vi "SaveData.vi"(1 "output cluster":cluster{"Position":dbl, "data":dbl[][]}, 3 "File name":string="radial.txt", 4 "File path":path=path "C:/Documents and Settings/Administrator/Desktop/labview/M_Coupling/radial_coupling") -> ()   [LabVIEW 2013]
panel:
  out "appended path":path
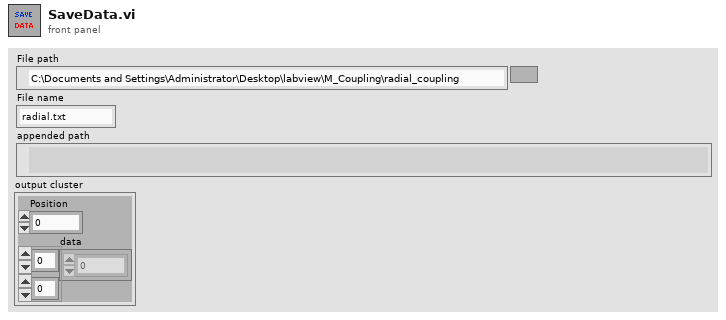
[diagram p1: front panel]
types:
  T1 = enum16{"open", "replace", "create", "open or create", "replace or create", "replace or create with confirmation"}
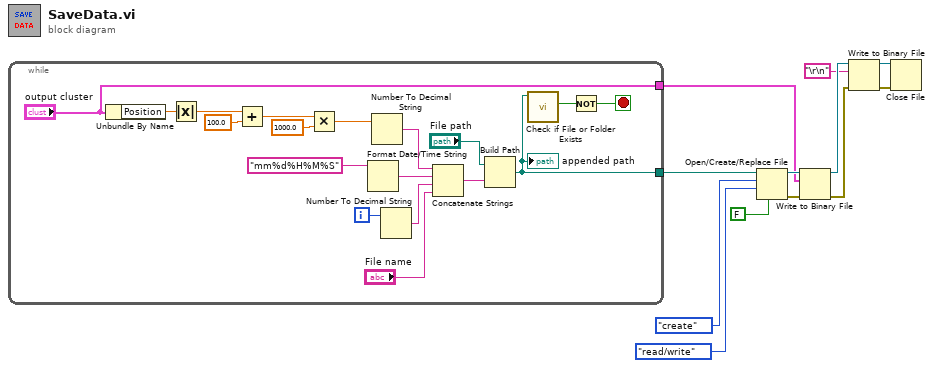
[diagram p0: block diagram]
diagram:
  n1 = while {
    tunnel: [w22] -> w7
    tunnel: ["output cluster"] -> w1
    i -> [w24]
    stop <- w26 stop-if-true
    n2 = Unbundle By Name("output cluster") -> ("Position"=w13:dbl)
    n3 = Absolute Value(x=w13) -> (abs(x)=w14:dbl)
    n4 = Add(x=w14, y=100.0) -> (x+y=w18:dbl)
    n5 = Multiply(x=w18, y=1000.0) -> (x*y=w16:dbl)
    n6 = Format Date/Time String(time format string (%c)="mm%d%H%M%S") -> (date/time string=w28:string)  [unwired: 2 in]
    n7 = Number To Decimal String(number=w16) -> (decimal integer string=w15:string)  [unwired: 1 in]
    n8 = Number To Decimal String(number=w24) -> (decimal integer string=w23:string)  [unwired: 1 in]
    n9 = Concatenate Strings(w15, w28, w23, "File name") -> (w27:string)
    n10 = Build Path(base path="File path", name or relative path=w27) -> (appended path=w22:path)
    "appended path" <- w22
    n11 = call <vilib>:"Check if File or Folder Exists.vi"("path"=w22) -> ("file or folder exists?"=w30:bool)  [unwired: 8 in, 2 out]
    n12 = Not(x=w30) -> (.not. x?=w26:bool)
  }
  n13 = Open/Create/Replace File(file path (use dialog)=w7, operation (0:open)=T1."create", access (0:read/write)=enum16{"read/write", "read-only", "write-only"}."read/write", disable buffering (F)=FALSE) -> (refnum out=w8:refnum<file>, error out=w9:errorcluster)  [unwired: 2 in, 1 out]
  n14 = Write to Binary File(file (use dialog)=w8, data=w1, error in=w9) -> (refnum out=w6:refnum<file>, error out=w5:errorcluster)  [unwired: 3 in, 1 out]
  n15 = Write to Binary File(file (use dialog)=w6, data="\r\n", error in=w5) -> (refnum out=w3:refnum<file>, error out=w4:errorcluster)  [unwired: 3 in, 1 out]
  n16 = Close File(refnum=w3, error in=w4) -> ()  [unwired: 2 out]
